vi "ShiftRegister.vi"() -> ()   [LabVIEW 2019]
panel:
  out "Previous Iteration":u16
  out "Current Iteration":u16
  in  "stop":bool
  out "Numeric":u16
  in  "a":u16
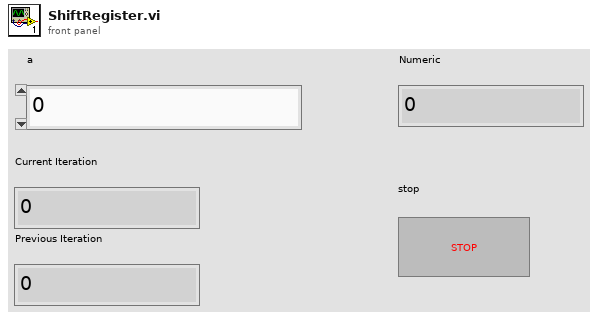
[diagram p1: front panel]
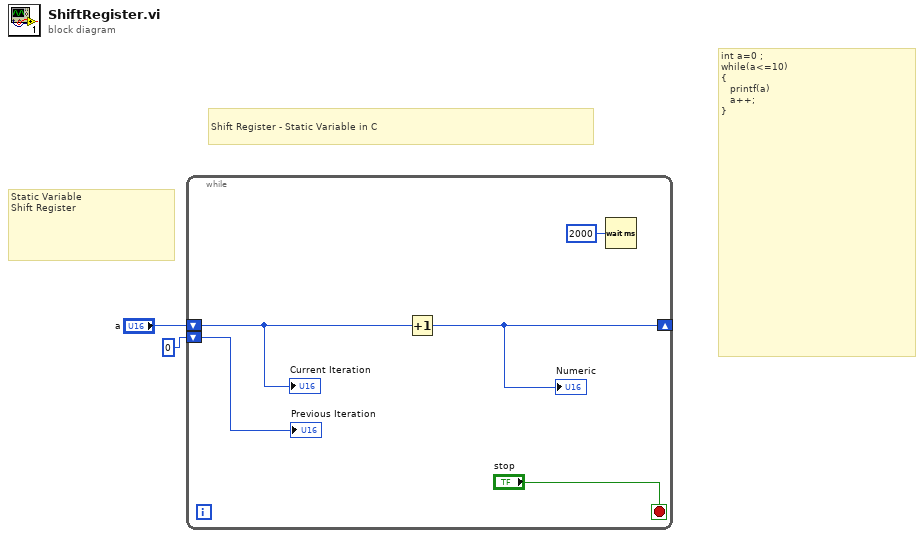
[diagram p0: block diagram]
diagram:
  # "Static Variable\nShift Register"
  # "Shift Register - Static Variable in C"
  # "int a=0 ;\nwhile(a<=10)\n{\n   printf(a)\n   a++; \n}"
  n1 = while {
    shift-right: [w7] -> _
    shift-left: "a" -> [w4]
    shift-left: u16 0 ("a") -> [w3]
    stop <- "stop" stop-if-true
    n2 = Increment(x=w4) -> (x+1=w7:u16)
    "Numeric" <- w7
    n3 = Wait (ms)(milliseconds to wait=u32 2000) -> ()  [unwired: 1 out]
    "Current Iteration" <- w4
    "Previous Iteration" <- w3
  }
